vi "Write FAMM-Queue.vi"(8 "error in (no error)":errorcluster, 10 "FAMM-Queue":refnum<queue>, 11 "FAMM in":refnum<class "FAMM.lvclass">) -> (0 "error out":errorcluster, 3 "FAMM out":refnum<class "FAMM.lvclass">)   [LabVIEW 2020, in "Sgraph_lib_V1.lvlib" / "FAMM.lvclass"]
uses:
  FAMM.lvclass
  controls/typedef_FAMM_Query.ctl
  controls/typedef-functions.ctl
  FAMM.lvclass/FAMM.ctl
  Builds/Sgraph_lib_V1.lvlib
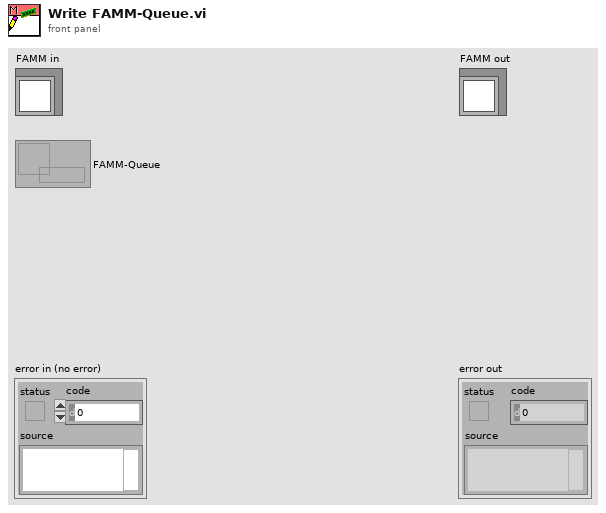
[diagram p1: front panel]
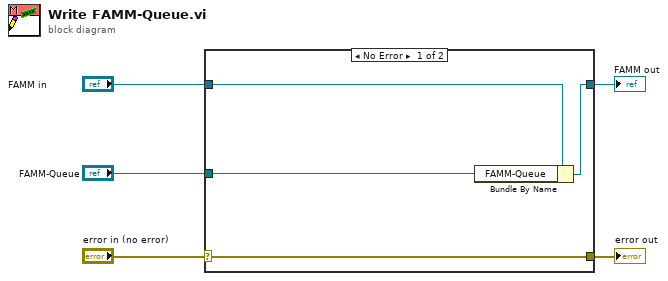
[diagram p0: block diagram]
diagram:
  n1 = case shown="No Error" "error in (no error)" {
    selector: "error in (no error)" -> [w9 w10]
    tunnel: [w9 w10] -> w4
    tunnel: [w7 w11] -> w2
    tunnel: "FAMM in" -> [w8 w11]
    tunnel: "FAMM-Queue" -> [w6 _]
    frame No Error {
      n2 = Bundle By Name(cluster=w8, "FAMM-Queue"=w6) -> (w7:refnum<class "FAMM.lvclass">)
    }
    frame Error {
    }
  }
  "error out" <- w4
  "FAMM out" <- w2
